vi "Test Waveforms.vi"(8 "error in (no error)":errorcluster, 11 "DAQmx in":refnum<class "DAQmx.lvclass">) -> (0 "error out":errorcluster, 2 "Waveforms":waveform(dbl)[](array[waveform]), 3 "DAQmx out":refnum<class "DAQmx.lvclass">)   [LabVIEW 2019, in "DAQmx.lvclass"]
uses:
  DAQmx.lvclass
  <vilib>/measure/NI_MABase.lvlib
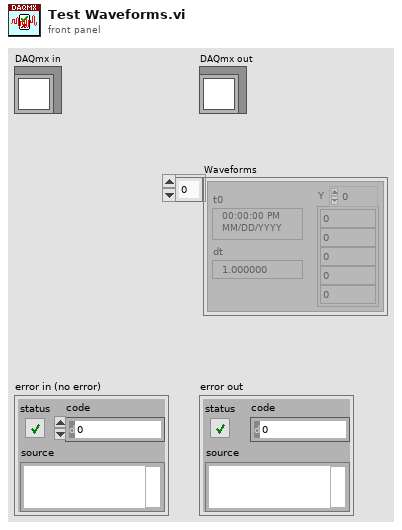
[diagram p1: front panel]
types:
  T1 = typedef "DAQmx.lvclass/DAQ.Config.Timing.Sampling--Cluster.ctl" = cluster{"Fs":dbl, "#s":i32}
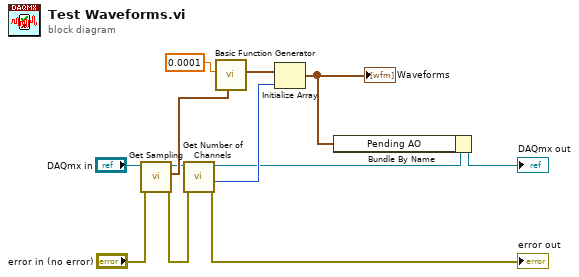
[diagram p0: block diagram]
diagram:
  n1 = call "Get Sampling.vi"("error in (no error)"="error in (no error)", "DAQmx in"="DAQmx in") -> ("error out"=w10:errorcluster, "Sampling info"=w12:T1, "DAQmx out"=w8:refnum<class "DAQmx.lvclass">)  [unwired: 7 in]
  n2 = call "Get Number of Channels.vi"("error in (no error)"=w10, "DAQmx in"=w8) -> ("error out"=→"error out":errorcluster, "Total Channels"=w5:u32, "DAQmx out"=w2:refnum<class "DAQmx.lvclass">)  [unwired: 6 in, 1 out]
  n3 = call <vilib>:"Basic Function Generator.vi"("sampling info"=w12, "amplitude"=0.0001) -> ("signal out"=w4:waveform(dbl))  [unwired: 7 in, 2 out]
  n4 = Initialize Array(w4, w5) -> (w3:waveform(dbl)[])
  "Waveforms" <- w3
  n5 = Bundle By Name(cluster=w2, "Pending AO"=w3) -> (→"DAQmx out":refnum<class "DAQmx.lvclass">)
